vi "PolymorphicSubVI reference.vi"() -> (0 "PolymorphicSubVI class constant":refnum<vi>)   [LabVIEW 2012, in "Scripting Tools.lvlib"]
uses:
  Scripting Tools.lvlib
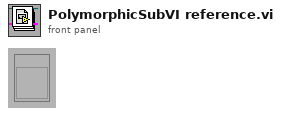
[diagram p1: front panel]
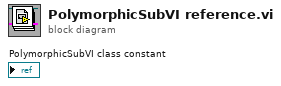
[diagram p0: block diagram]
diagram:
